vi "UniversalExtract.vi"(5 "Input Array":string[][](array[string]), 11 "Error In":errorcluster) -> (6 "Data Parameters":T1(array[cluster]), 10 "PLC cluster":T2, 15 "Error Out":errorcluster)   [LabVIEW 2014]
uses:
  Controls/ColumnHeaders1.ctl
  <userlib>/_RADE/MTA-lib/array/array.llb/Remove Duplicates from 1D Array (String)__ogtk.vi
panel:
  out "Array":string[](array[string])
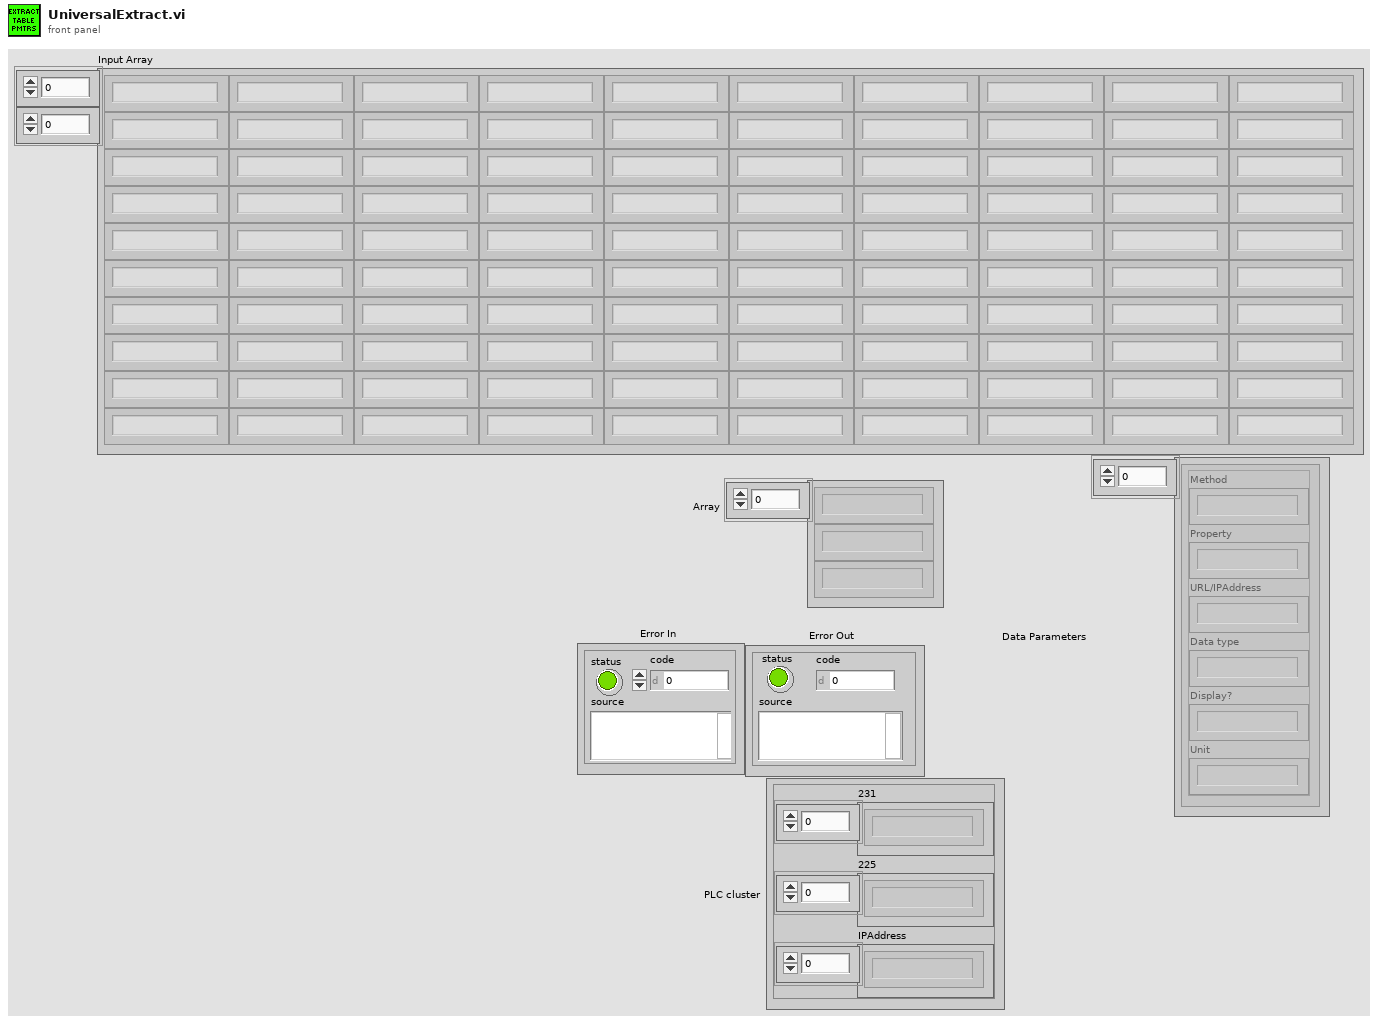
[diagram p1: front panel]
types:
  T1 = cluster{"Method":string, "Property":string, "URL/IPAddress":string, "Data type":string, "Display?":string, "Unit":string}[]
  T2 = cluster{"231":string[], "225":string[], "IPAddress":string[]}
  T3 = typedef "ColumnHeaders1.ctl" = enum16{"Store", "Display", "Method", "Property", "Unit", "URL", "IP Address", "Data Block", "Address", "Data Type"}
  T4 = cluster{"String":string, "String":string, "String":string, "String":string, "String":string, "String":string}[]
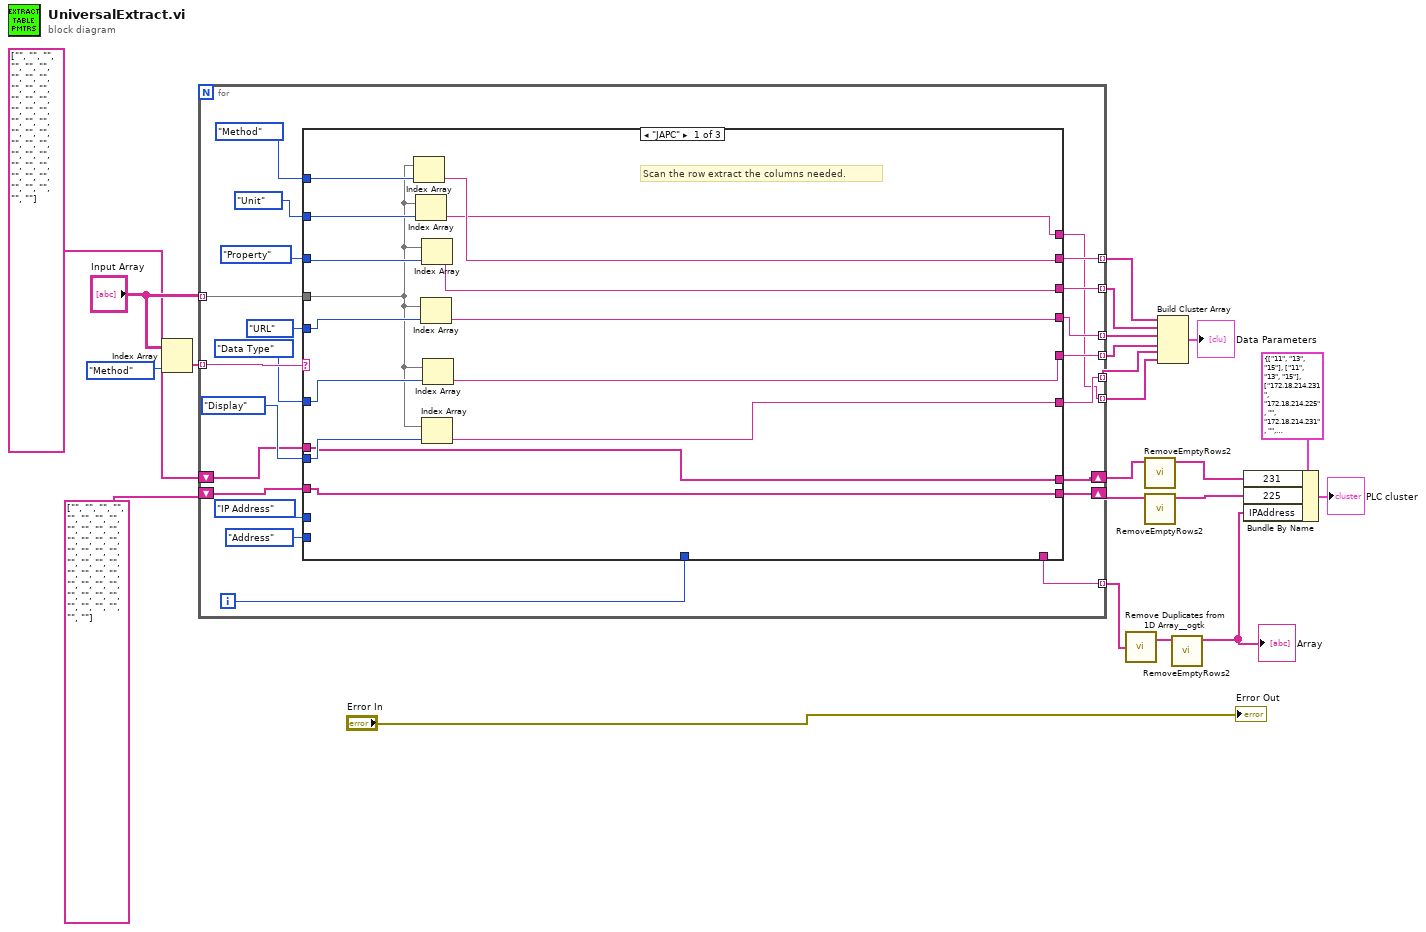
[diagram p0: block diagram]
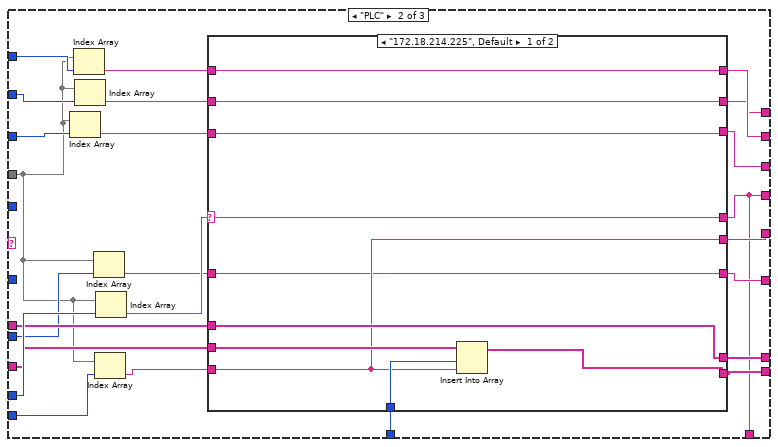
[diagram p2: hidden frame]
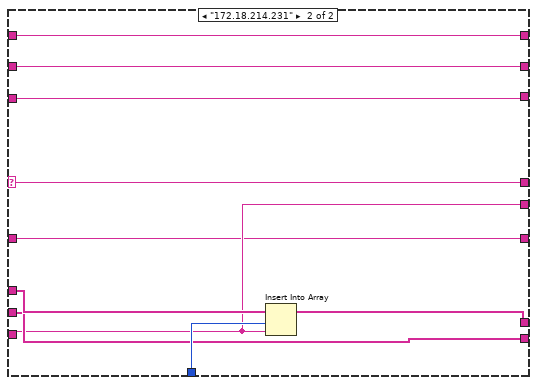
[diagram p3: hidden frame]
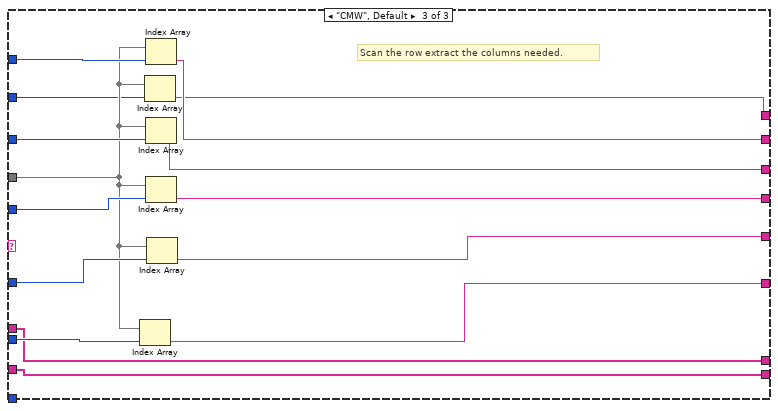
[diagram p4: hidden frame]
diagram:
  n1 = Index Array(array="Input Array", index (col)=ColumnHeaders1."Method" ("ColumnHeaders")) -> (element=w14:string[])  [unwired: 1 in]
  n2 = for {
    tunnel: w14 -> [w44] mode=indexing
    tunnel: "Input Array" -> [w43] mode=indexing
    tunnel: [w42] -> w20 mode=indexing
    tunnel: [w41] -> w19 mode=indexing
    tunnel: [w26] -> w18 mode=indexing
    tunnel: [w40] -> w17 mode=indexing
    tunnel: [w27] -> w16 mode=indexing
    shift-right: [w31] -> w11
    shift-left: string[] ["", "", "", "", "", "", "", "", "", "", "", "", "", "", "", "", "", "", "", "", "", "", "", "", "", "", "", "", "", "", "", "", "", "", "", "", "", "", "", "", ""] -> [w30]
    shift-right: [w28] -> w10
    shift-left: string[] ["", "", "", "", "", "", "", "", "", "", "", "", "", "", "", "", "", "", "", "", "", "", "", "", "", "", "", "", "", "", "", "", "", "", "", "", "", "", "", "", "", ""] -> [w29]
    tunnel: [w25] -> w6 mode=indexing
    tunnel: [w23] -> w2 mode=indexing
    i -> [w32]
    n3 = case shown="\"JAPC\"" w44 {
      tunnel: w43 -> [w46 w61 w106]
      tunnel: [w59 w69 w118] -> w42
      tunnel: [w58 w70 w117] -> w41
      tunnel: [w57 w64 w116] -> w26
      tunnel: [w56 w68 w115] -> w40
      tunnel: [w55 w65 w114] -> w27
      tunnel: ColumnHeaders1."Display" ("Display?") -> [w50 w67 w113]
      tunnel: ColumnHeaders1."Data Type" ("Data Type") -> [w51 _ w112]
      tunnel: ColumnHeaders1."Method" ("Method") -> [w54 w72 w111]
      tunnel: ColumnHeaders1."Property" ("Property") -> [w53 w74 w110]
      tunnel: ColumnHeaders1."URL" ("URL") -> [w52 _ w109]
      tunnel: ColumnHeaders1."IP Address" ("IP Address") -> [_ w83 _]
      tunnel: ColumnHeaders1."Address" ("Address") -> [_ w81 _]
      tunnel: [w48 w79 w107] -> w28
      tunnel: [w49 w78 w108] -> w31
      tunnel: w32 -> [_ w77 _]
      tunnel: w30 -> [w49 w76 w108]
      tunnel: w29 -> [w48 w75 w107]
      tunnel: [_ w64 _] -> w25
      tunnel: ColumnHeaders1."Unit" ("Method") -> [w47 w63 w105]
      tunnel: [w45 w60 w104] -> w23
      frame "JAPC" {
        # "Scan the row extract the columns needed."
        n4 = Index Array(array=w46, index=w54) -> (element=w59:string)
        n5 = Index Array(array=w46, index=w47) -> (element=w45:string)
        n6 = Index Array(array=w46, index=w52) -> (element=w57:string)
        n7 = Index Array(array=w46, index=w53) -> (element=w58:string)
        n8 = Index Array(array=w46, index=w50) -> (element=w55:string)
        n9 = Index Array(array=w46, index=w51) -> (element=w56:string)
      }
      frame "PLC" {
        n10 = Index Array(array=w61, index=w74) -> (element=w73:string)
        n11 = Index Array(array=w61, index=w72) -> (element=w71:string)
        n12 = Index Array(array=w61, index=w63) -> (element=w62:string)
        n13 = Index Array(array=w61, index=w67) -> (element=w66:string)
        n14 = Index Array(array=w61, index=w81) -> (element=w80:string)
        n15 = Index Array(array=w61, index=w83) -> (element=w82:string)
        n16 = case shown="\"172.18.214.225\", Default" w82 {
          selector: w82 -> [w86 w97]
          tunnel: w80 -> [w87 w96]
          tunnel: [w93 w100] -> w79
          tunnel: [w90 w103] -> w78
          tunnel: w77 -> [w92 w102]
          tunnel: w76 -> [w90 w101]
          tunnel: w75 -> [w91 w100]
          tunnel: w73 -> [w88 w98]
          tunnel: w71 -> [w89 w99]
          tunnel: [w89 w99] -> w69
          tunnel: [w88 w98] -> w70
          tunnel: [w86 w97] -> w64
          tunnel: [w87 w96] -> w68
          tunnel: w66 -> [w85 w95]
          tunnel: [w85 w95] -> w65
          tunnel: w62 -> [w84 w94]
          tunnel: [w84 w94] -> w60
          frame "172.18.214.225", Default {
            n17 = Insert Into Array(array=w91, index=w92, new element=w87) -> (w93:string[])
          }
          frame "172.18.214.231" {
            n18 = Insert Into Array(array=w101, index=w102, new element=w96) -> (w103:string[])
          }
        }
      }
      frame "CMW", Default {
        # "Scan the row extract the columns needed."
        n19 = Index Array(array=w106, index=w113) -> (element=w114:string)
        n20 = Index Array(array=w106, index=w105) -> (element=w104:string)
        n21 = Index Array(array=w106, index=w111) -> (element=w118:string)
        n22 = Index Array(array=w106, index=w110) -> (element=w117:string)
        n23 = Index Array(array=w106, index=w109) -> (element=w116:string)
        n24 = Index Array(array=w106, index=w112) -> (element=w115:string)
      }
    }
  }
  n25 = call-poly <userlib>:"Remove Duplicates from 1D Array__ogtk.vi"("Input Array"=w6) -> ("Output Array"=w4:string[])  [unwired: 1 out]
  n26 = call "RemoveEmptyRows2.vi"("Array 3"=w11) -> ("Array 4"=w8:string[])  [unwired: 9 in, 1 out]
  n27 = call "RemoveEmptyRows2.vi"("Array 3"=w10) -> ("Array 4"=w7:string[])  [unwired: 9 in, 1 out]
  n28 = Build Cluster Array(w20, w19, w18, w17, w16, w2) -> (→"Data Parameters":T4)
  n29 = call "RemoveEmptyRows2.vi"("Array 3"=w4) -> ("Array 4"=w3:string[])  [unwired: 9 in, 1 out]
  "Array" <- w3
  n30 = Bundle By Name(cluster=T2 {"231"=["11", "13", "15"], "225"=["11", "13", "15"], "IPAddress"=["172.18.214.231", "172.18.214.225", "", "172.18.214.231", "", "172.18.214.225", "172.18.214.231"]} ("input cluster"), "231"=w8, "225"=w7, "IPAddress"=w3) -> (→"PLC cluster":T2)
  "Error Out" <- "Error In"
